vi "Remove OBJ Tag.vi"(11 "Name":string) -> (2 "tagged as Item Name in JSON Objects":bool, 3 "Name (tag stripped)":string)   [LabVIEW 2019, in "JSONtext.lvlib"]
uses:
  JSONtext.lvlib
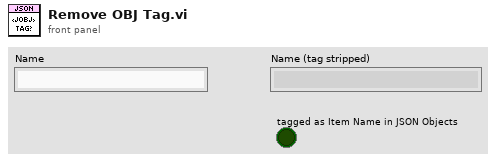
[diagram p1: front panel]
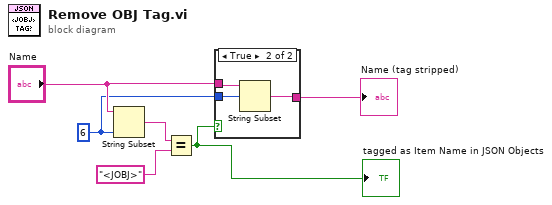
[diagram p0: block diagram]
diagram:
  w1 = 6 ("length (rest)")
  n1 = String Subset(string="Name", length (rest)=w1) -> (substring=w3:string)  [unwired: 1 in]
  n2 = Equal?(x=w3, y="<JOBJ>") -> (x = y?=w6:bool)
  "tagged as Item Name in JSON Objects" <- w6
  n3 = case shown="True" w6 {
    tunnel: [w7 w9] -> w4
    tunnel: "Name" -> [w7 w10]
    tunnel: w1 -> [_ w8]
    frame False {
    }
    frame True {
      n4 = String Subset(string=w10, offset (0)=w8) -> (substring=w9:string)  [unwired: 1 in]
    }
  }
  "Name (tag stripped)" <- w4
